vi "Get Child.vi"(6 "Index in":i32, 8 "error in (no error)":errorcluster, 11 "Composite Object in":refnum<class "CConfig Object.lvclass">) -> (0 "error out":errorcluster, 2 "Child":refnum<class "CConfig Object.lvclass">, 3 "Composite Object out":refnum<class "CConfig Object.lvclass">)   [LabVIEW 2013, in "CConfig Object.lvclass"]
doc: "Copyright 2018, Carya Automatisering, Wiebe Walstra."
uses:
  CConfig Object.lvclass
  CConfig Object.lvclass/CConfig Object.ctl
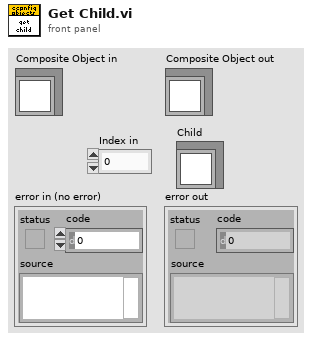
[diagram p1: front panel]
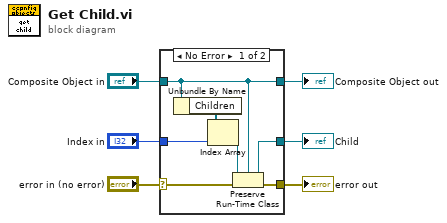
[diagram p0: block diagram]
diagram:
  n1 = case shown="No Error" "error in (no error)" {
    selector: "error in (no error)" -> [w8 w15]
    tunnel: [w7 w15] -> w5
    tunnel: [w9 w14] -> w3
    tunnel: "Composite Object in" -> [w9 w14]
    tunnel: "Index in" -> [w13 _]
    tunnel: [w10 _] -> w1
    frame No Error {
      n2 = Unbundle By Name(w9) -> ("Children"=w12:refnum<class>[])
      n3 = Index Array(array=w12, index=w13) -> (element=w11:refnum<class>)
      n4 = Preserve Run-Time Class(object in=w11, error in=w8, 2:w9) -> (object out=w10:refnum<class "CConfig Object.lvclass">, error out=w7:errorcluster)
    }
    frame Error {
    }
  }
  "error out" <- w5
  "Composite Object out" <- w3
  "Child" <- w1
